vi "Voronoi_Main.vi"(9 "Triangles":i32[][](array[numeric]), 10 "Y":dbl[](array[numeric]), 11 "X":dbl[](array[numeric])) -> (2 "Edge Y":dbl[][](array[numeric]), 3 "Edge X":dbl[][](array[numeric]))   [LabVIEW 2017, in "NI_AAL_Geometry.lvlib"]
uses:
  <vilib>/Analysis/NI_AAL_Geometry.lvlib
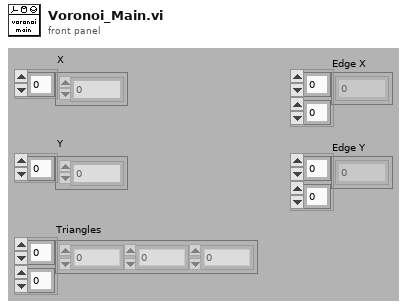
[diagram p1: front panel]
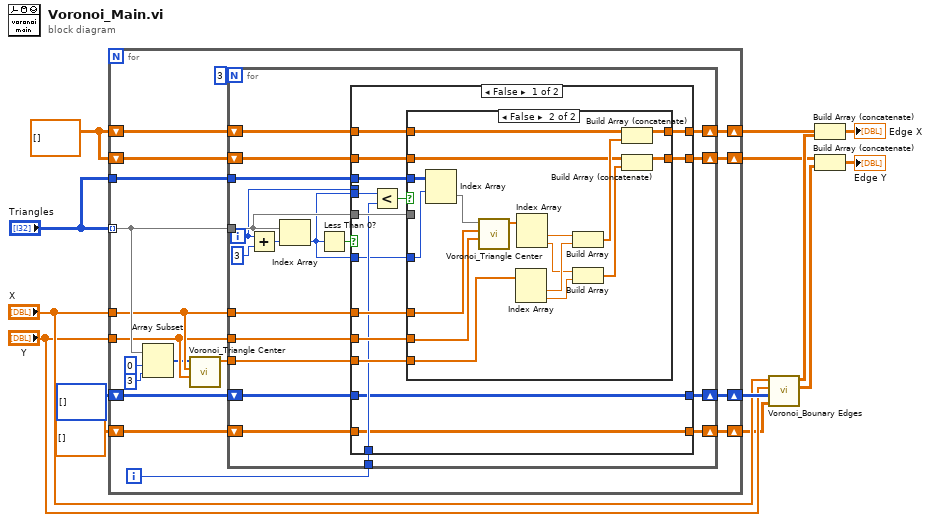
[diagram p0: block diagram]
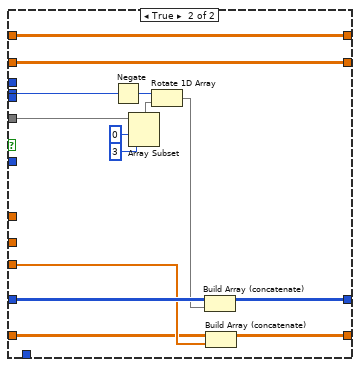
[diagram p3: hidden frame]
diagram:
  w14 = dbl[][] []
  n1 = for {
    tunnel: "Triangles" -> [w32] mode=indexing
    tunnel: "X" -> [w30]
    tunnel: "Y" -> [w29]
    shift-right: [w26] -> w6
    shift-left: w14 -> [w27]
    shift-right: [w25] -> w3
    shift-left: w14 -> [w28]
    tunnel: "Triangles" -> [w19]
    shift-right: [w17] -> w11
    shift-left: i32[][] [] -> [w18]
    shift-right: [w15] -> w7
    shift-left: dbl[][] [] -> [w16]
    i -> [w31]
    n2 = Array Subset(array=w32, index=0, length=3) -> (w21:i32[])
    n3 = call <vilib>:"Voronoi_Triangle Center.vi"("Y"=w29, "X"=w30, "Triangle"=w21) -> ("Delaunay Center"=w20:dbl[])  [unwired: 8 in]
    n4 = for {
      N: 3 -> [_]
      tunnel: w32 -> [w42]
      tunnel: w31 -> [w40]
      tunnel: w30 -> [w50]
      tunnel: w29 -> [w49]
      tunnel: w20 -> [w48]
      shift-right: [w44] -> w25
      shift-left: w28 -> [w47]
      shift-right: [w45] -> w26
      shift-left: w27 -> [w46]
      tunnel: w19 -> [w39]
      shift-right: [w35] -> w17
      shift-left: w18 -> [w36]
      shift-right: [w33] -> w15
      shift-left: w16 -> [w34]
      i -> [w41]
      n5 = Add(x=w41, y=3) -> (x+y=w38:i32)
      n6 = Index Array(array=w42, index=w38) -> (element=w37:i32)
      n7 = Less Than 0?(x=w37) -> (x < 0?=w43:bool)
      n8 = case shown="False" w43 {
        tunnel: w42 -> [w66 w99]
        tunnel: w50 -> [w65 _]
        tunnel: w49 -> [w64 _]
        tunnel: w48 -> [w63 w89]
        tunnel: w47 -> [w60 w92]
        tunnel: w46 -> [w61 w93]
        tunnel: [w62 w93] -> w45
        tunnel: [w59 w92] -> w44
        tunnel: w41 -> [_ w95]
        tunnel: w37 -> [w58 _]
        tunnel: w40 -> [w57 _]
        tunnel: w39 -> [w55 _]
        tunnel: w37 -> [w54 _]
        tunnel: w36 -> [w53 w91]
        tunnel: [w53 w90] -> w35
        tunnel: w34 -> [w52 w88]
        tunnel: [w52 w87] -> w33
        frame False {
          n9 = Less?(x=w58, y=w57) -> (x < y?=w56:bool)
          n10 = case shown="False" w56 {
            tunnel: w66 -> [_ _]
            tunnel: w65 -> [_ w85]
            tunnel: w64 -> [_ w84]
            tunnel: w63 -> [_ w82]
            tunnel: [w68 w77] -> w62
            tunnel: w61 -> [w68 w76]
            tunnel: w60 -> [w67 w73]
            tunnel: [w67 w72] -> w59
            tunnel: w55 -> [_ w71]
            tunnel: w54 -> [_ w70]
            frame True {
            }
            frame False {
              n11 = Index Array(array=w71, index (row)=w70) -> (element=w69:i32[])  [unwired: 1 in]
              n12 = call <vilib>:"Voronoi_Triangle Center.vi"("Y"=w84, "X"=w85, "Triangle"=w69) -> ("Delaunay Center"=w83:dbl[])  [unwired: 8 in]
              n13 = Index Array(array=w82) -> (element #1=w80:dbl, element #2=w78:dbl)  [unwired: 2 in]
              n14 = Index Array(array=w83) -> (element #1=w81:dbl, element #2=w79:dbl)  [unwired: 2 in]
              n15 = Build Array(w81, w80) -> (w75:dbl[])
              n16 = Build Array(w79, w78) -> (w74:dbl[])
              n17 = Build Array (concatenate)(w76, w75) -> (w77:dbl[][])
              n18 = Build Array (concatenate)(w73, w74) -> (w72:dbl[][])
            }
          }
        }
        frame True {
          n19 = Negate(x=w95) -> (-x=w94:i32)
          n20 = Array Subset(array=w99, index=0, length=3) -> (w96:i32[])
          n21 = Rotate 1D Array(1:w96, 2:w94) -> (0:w86:i32[])
          n22 = Build Array (concatenate)(w91, w86) -> (w90:i32[][])
          n23 = Build Array (concatenate)(w88, w89) -> (w87:dbl[][])
        }
      }
    }
  }
  n24 = call <vilib>:"Voronoi_Bounary Edges.vi"("Centers"=w7, "Triangles"=w11, "Y"="Y", "X"="X") -> ("Edge Y"=w2:dbl[][], "Edge X"=w5:dbl[][])  [unwired: 6 in]
  n25 = Build Array (concatenate)(w6, w5) -> (→"Edge X":dbl[][])
  n26 = Build Array (concatenate)(w3, w2) -> (→"Edge Y":dbl[][])
